vi "CreateTriggerChannelNode.vi"(7 "DOM Document":refnum<k20>, 8 "Error In":errorcluster, 11 "Trigger Channel Configuration":T1) -> (0 "Error Out":errorcluster, 3 "Trigger Channel Node":refnum<k20>)   [LabVIEW 2012]
uses:
  TriggerChannelConfiguration.ctl
  driver/Public/Controls/TriggerSource.ctl
  libs/LV-Utilities/LV-Utilities.lvlib
  driver/Keithley-7001.lvlib
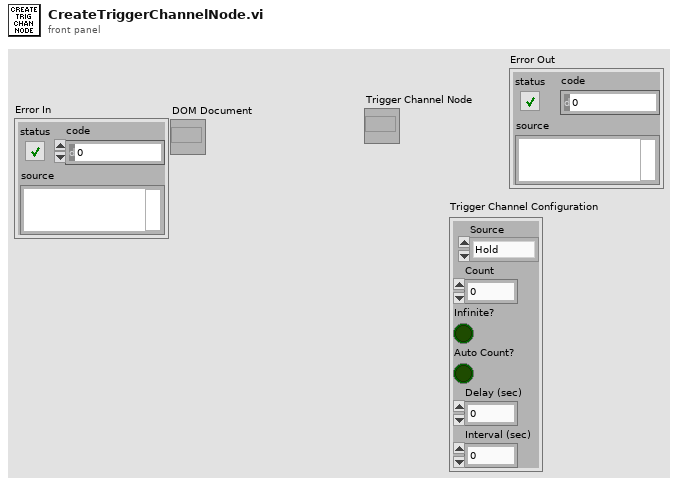
[diagram p1: front panel]
types:
  T1 = typedef "TriggerChannelConfiguration.ctl" = cluster{"Source":T2, "Count":u32, "Infinite?":bool, "Auto Count?":bool, "Delay (sec)":dbl, "Interval (sec)":dbl}
  T2 = typedef "Keithley-7001.lvlib/TriggerSource.ctl" = enum16{"Hold", "Immediate", "Manual", "Bus", "TLink", "External", "Timer"}
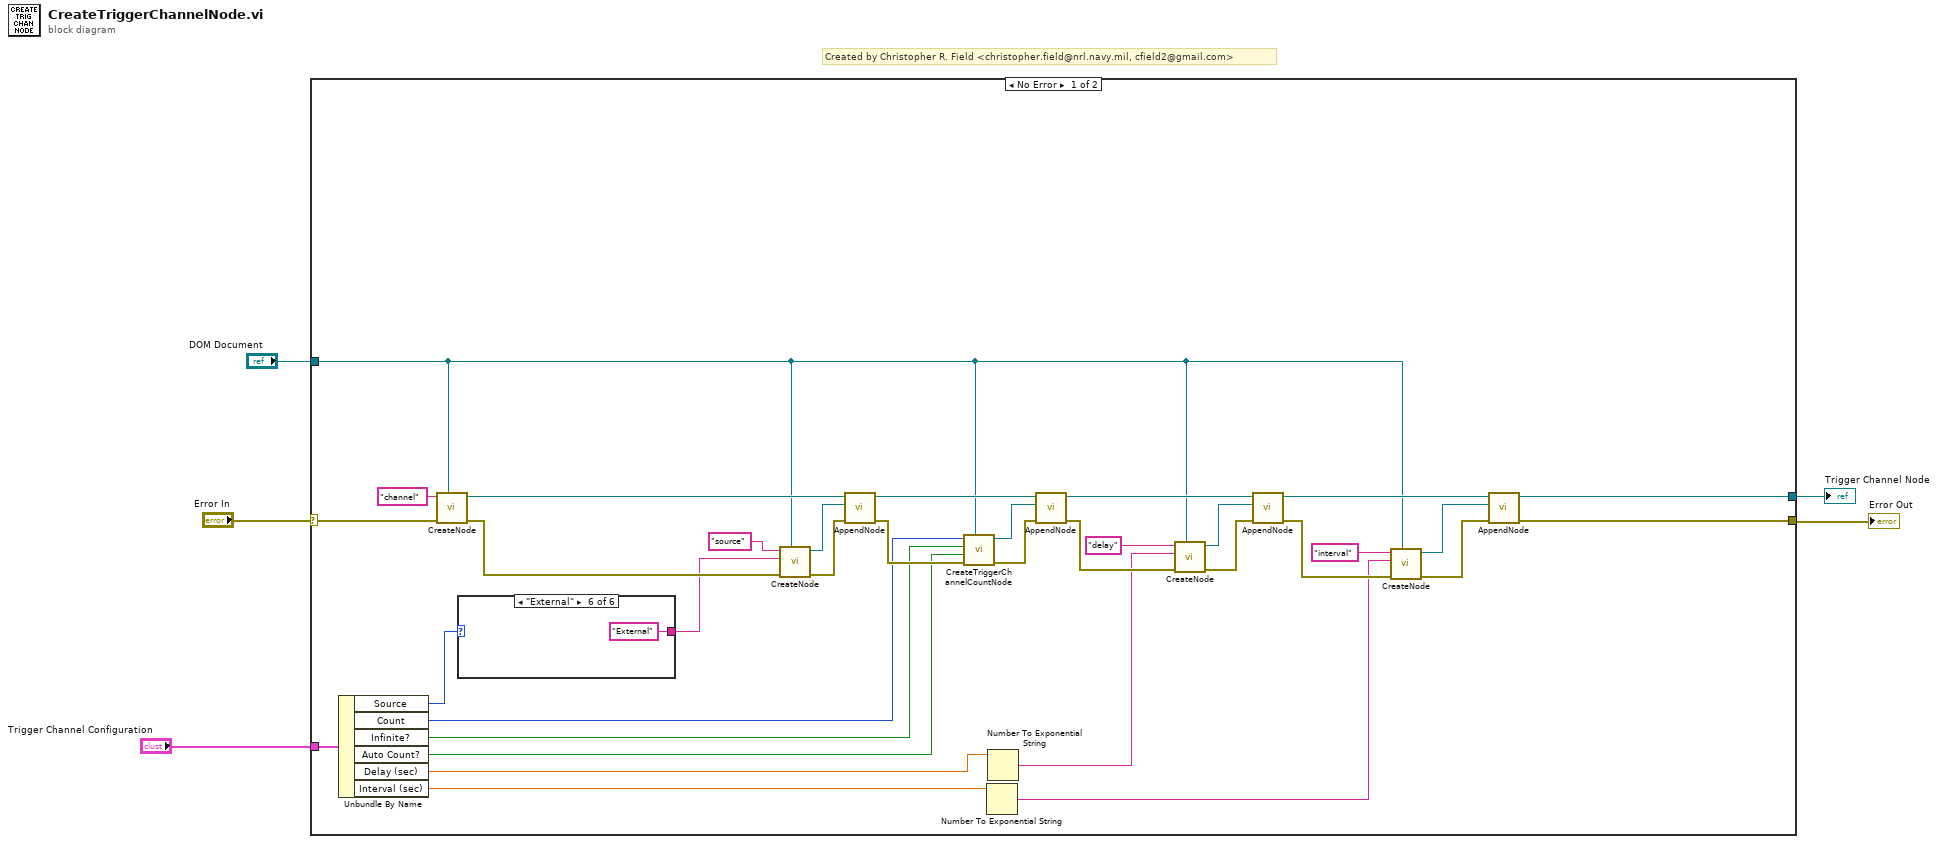
[diagram p0: block diagram]
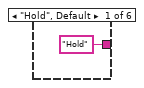
[diagram p2: hidden frame]
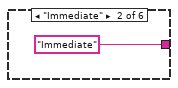
[diagram p3: hidden frame]
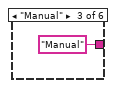
[diagram p4: hidden frame]
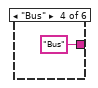
[diagram p5: hidden frame]
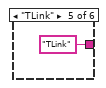
[diagram p6: hidden frame]
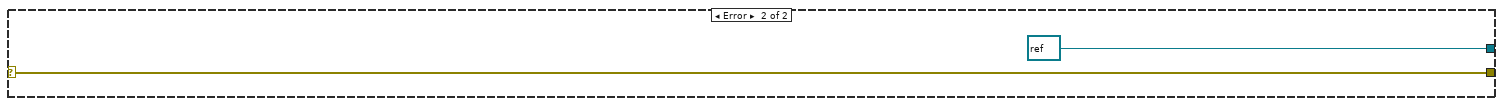
[diagram p7: hidden frame]
diagram:
  # "Created by Christopher R. Field <christopher.field@nrl.navy.mil, cfield2@gmail.com>"
  n1 = case shown="No Error" "Error In" {
    selector: "Error In" -> [w39 w47]
    tunnel: "DOM Document" -> [w12 _]
    tunnel: [w14 w47] -> w3
    tunnel: [w15 refnum<k20> refnum ("Wirings Node 2")] -> w2
    tunnel: "Trigger Channel Configuration" -> [w32 _]
    frame No Error {
      n2 = Unbundle By Name(w32) -> ("Source"=w31:T2, "Count"=w10:u32, "Infinite?"=w9:bool, "Auto Count?"=w8:bool, "Delay (sec)"=w13:dbl, "Interval (sec)"=w22:dbl)
      n3 = call "CreateNode.vi"("DOM Document"=w12, "Error In"=w39, "Tag Name"="channel") -> ("Error out"=w36:errorcluster, "Node"=w35:refnum<k20>)  [unwired: 7 in]
      n4 = case shown="\"External\"" w31 {
        tunnel: ["Hold" "Immediate" "Manual" "Bus" "TLink" "External"] -> w30
        frame "Hold", Default {
        }
        frame "Immediate" {
        }
        frame "Manual" {
        }
        frame "Bus" {
        }
        frame "TLink" {
        }
        frame "External" {
        }
      }
      n5 = call "CreateNode.vi"("DOM Document"=w12, "Error In"=w36, "Text"=w30, "Tag Name"="source") -> ("Error out"=w34:errorcluster, "Node"=w33:refnum<k20>)  [unwired: 6 in]
      n6 = call "AppendNode.vi"("Error In"=w34, "Child Node"=w33, "Parent Node In"=w35) -> ("Error Out"=w11:errorcluster, "Parent Node Out"=w29:refnum<k20>)  [unwired: 7 in]
      n7 = call "CreateTriggerChannelCountNode.vi"("DOM Document"=w12, "Error In"=w11, "Auto Count?"=w8, "Infinite?"=w9, "Count"=w10) -> ("Error Out"=w7:errorcluster, "Trigger Channel Count Node"=w6:refnum<k20>)  [unwired: 5 in]
      n8 = Number To Exponential String(number=w22) -> (E-format string=w20:string)  [unwired: 3 in]
      n9 = Number To Exponential String(number=w13) -> (E-format string=w27:string)  [unwired: 3 in]
      n10 = call "AppendNode.vi"("Error In"=w7, "Child Node"=w6, "Parent Node In"=w29) -> ("Error Out"=w28:errorcluster, "Parent Node Out"=w25:refnum<k20>)  [unwired: 7 in]
      n11 = call "CreateNode.vi"("DOM Document"=w12, "Error In"=w28, "Text"=w27, "Tag Name"="delay") -> ("Error out"=w23:errorcluster, "Node"=w24:refnum<k20>)  [unwired: 6 in]
      n12 = call "AppendNode.vi"("Error In"=w23, "Child Node"=w24, "Parent Node In"=w25) -> ("Error Out"=w21:errorcluster, "Parent Node Out"=w18:refnum<k20>)  [unwired: 7 in]
      n13 = call "CreateNode.vi"("DOM Document"=w12, "Error In"=w21, "Text"=w20, "Tag Name"="interval") -> ("Error out"=w17:errorcluster, "Node"=w16:refnum<k20>)  [unwired: 6 in]
      n14 = call "AppendNode.vi"("Error In"=w17, "Child Node"=w16, "Parent Node In"=w18) -> ("Error Out"=w14:errorcluster, "Parent Node Out"=w15:refnum<k20>)  [unwired: 7 in]
    }
    frame Error {
    }
  }
  "Trigger Channel Node" <- w2
  "Error Out" <- w3
